vi "GetSlideReference.vi"(8 "error in":errorcluster, 11 "Slide in":refnum<class "Slide.lvclass">) -> (0 "error out":errorcluster, 1 "slide reference":refnum<vi>, 3 "Slide out":refnum<class "Slide.lvclass">)   [LabVIEW 2014, in "Slide.lvclass"]
uses:
  Slide.lvclass
  Generic/Generic.lvclass
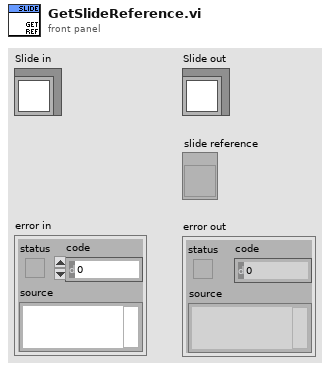
[diagram p1: front panel]
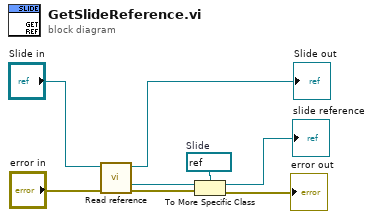
[diagram p0: block diagram]
diagram:
  w2 = refnum<vi> refnum  # Slide
  n1 = call "Read reference.vi"("error in"="error in", "GObject in"="Slide in") -> ("error out"=w6:errorcluster, "reference"=w5:refnum<vi>, "GObject out"=→"Slide out":refnum<class "Slide.lvclass">)  [unwired: 5 in]
  n2 = To More Specific Class(target class=w2, reference=w5, error in=w6) -> (specific class reference=→"slide reference":refnum<vi>, error out=→"error out":errorcluster)
